vi "test NtripClient_mount point only.vi"() -> ()   [LabVIEW 2019]
uses:
  Ctrl/Ntrip_Account_db.ctl
panel:
  out "에러 출력 2":errorcluster caption="에러 출력"
  in  "탭 컨트롤":enum32{"Main", "ref", "wireshark capture"}(tab)
  in  "Mount points":u16(ring) items=["SONP-RTCM32", "GANS-RTCM32", "GUMC-RTCM32", "DBON-RTCM32", "YONS-RTCM23", "SONP-RTCM23", "GUMC-RTCM23", "GANS-RTCM31", "YONS-CMRx", "SONP-RTCM31", "GUMC-RTCM31", "GANS-RTCM23", "DBON-RTCM23", "DBON-RTCM31", "YONS-RTCM31", "YONS-RTCM32-M5", "VRS-RTCM32-M5", "VRS-RTCM31", "VRS-CMRx", "VRS-CMRplus"]
  out "mount points":string[](array[string])
  out "링 텍스트.텍스트":string
  in  "Current Ntrip account":T1={"address"="gnss.eseoul.go.kr", "port "=2101, "id"="seoul", "pwd"="seoul", "ref pt"="YONS-RTCM32-M5"}
  in  "read bytes":i32=10000
  out "데이터 출력":string
  out "s? t:f":string
  # "fkp.ngii.go.kr"
  # "Test Ntrip Client"
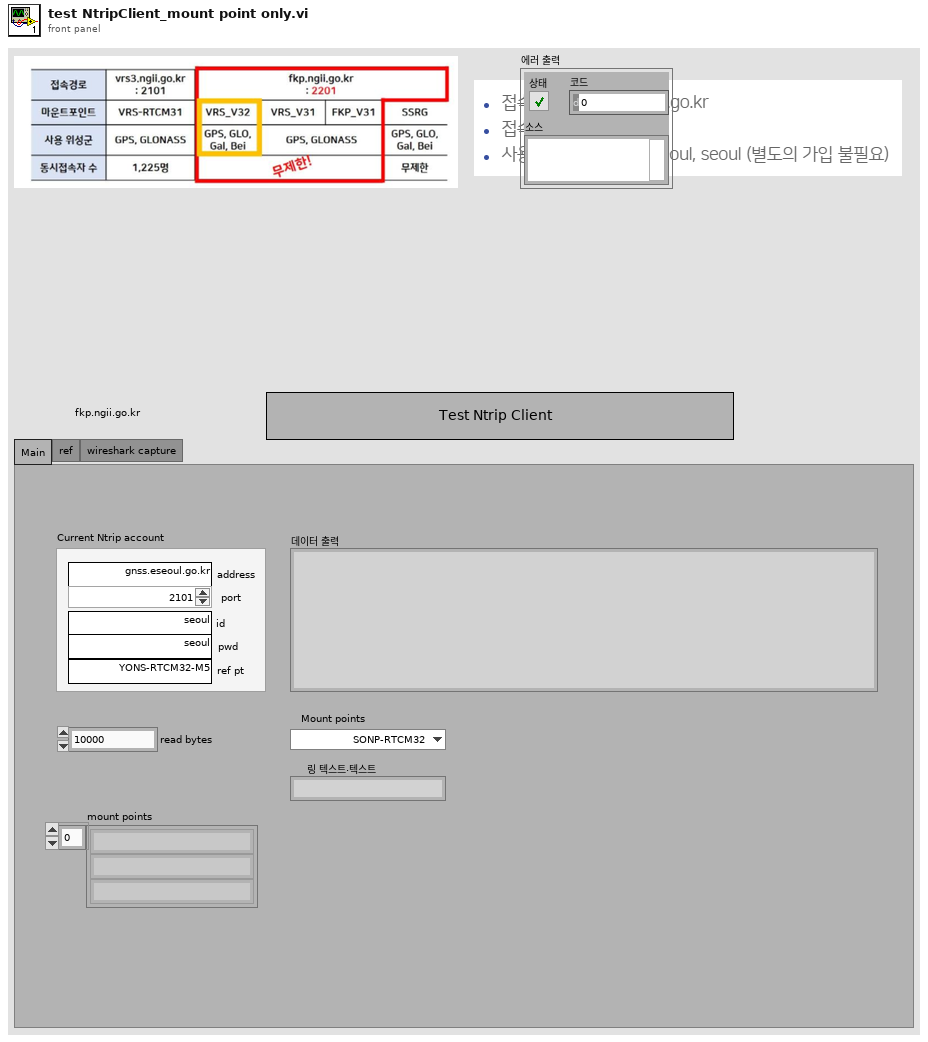
[diagram p1: front panel]
types:
  T1 = typedef "Ntrip_Account_db.ctl" = cluster{"address":string, "port ":u16, "id":string, "pwd":string, "ref pt":string}
  T2 = enum16{"Standard", "Buffered", "CRLF", "Immediate"}
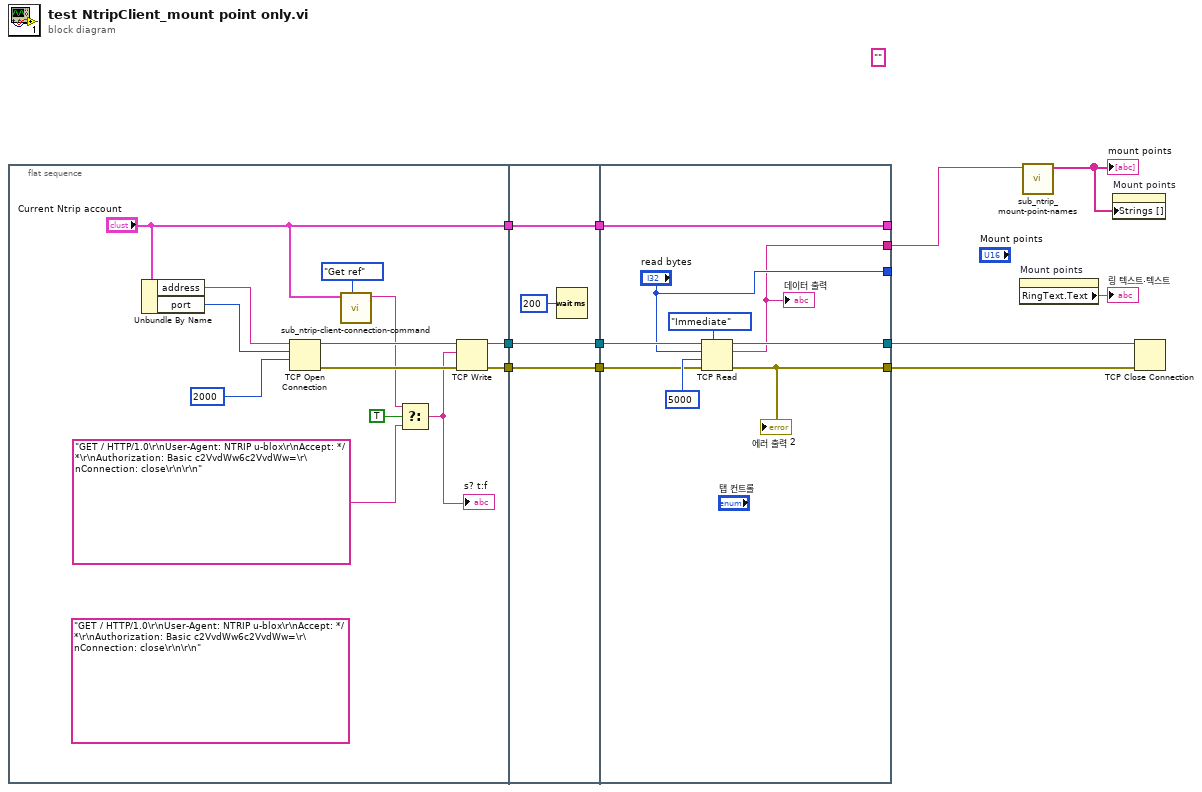
[diagram p0: block diagram]
diagram:
  (unwired) ""
  n1 = flat-sequence {
    tunnel: [w22] -> w11
    tunnel: [w21] -> w10
    tunnel: ["Current Ntrip account"] -> w9
    tunnel: w11 -> [w28]
    tunnel: w10 -> [w27]
    tunnel: w9 -> [w25]
    tunnel: [w28] -> w8
    tunnel: [w27] -> w7
    tunnel: [w25] -> w6
    tunnel: [w37] -> _
    tunnel: [w34] -> w5
    tunnel: [w31] -> w4
    tunnel: w8 -> [w32]
    tunnel: w7 -> [w33]
    tunnel: w6 -> [w37]
    tunnel: ["read bytes"] -> _
    tunnel: [w29] -> w1
    frame #0 {
      (unwired) "GET / HTTP/1.0\r\nUser-Agent: NTRIP u-blox\r\nAccept: */*\r\nAuthorization: Basic c2VvdWw6c2VvdWw=\r\nConnection: close\r\n\r\n" ("ascii 2")
      n2 = Unbundle By Name("Current Ntrip account") -> ("address"=w18:string, "port"=w17:u16)
      n3 = TCP Open Connection(address=w18, remote port or service name=w17, timeout ms (60000)=2000) -> (connection ID=w23:refnum<k5>, error out=w20:errorcluster)  [unwired: 2 in]
      n4 = call "sub_ntrip-client-connection-command.vi"("cmd"=enum16{"Get ref", "Get rtcm"}."Get ref", "Current Ntrip account"="Current Ntrip account") -> ("hex"=w14:string)  [unwired: 9 in]
      n5 = Select(t=w14, s=TRUE, f="GET / HTTP/1.0\r\nUser-Agent: NTRIP u-blox\r\nAccept: */*\r\nAuthorization: Basic c2VvdWw6c2VvdWw=\r\nConnection: close\r\n\r\n" ("ascii 2")) -> (s? t:f=w12:string)
      "s? t:f" <- w12
      n6 = TCP Write(connection ID=w23, data in=w12, error in (no error)=w20) -> (connection ID out=w21:refnum<k5>, error out=w22:errorcluster)  [unwired: 1 in, 1 out]
    }
    frame #1 {
      n7 = Wait (ms)(milliseconds to wait=u32 200) -> ()  [unwired: 1 out]
    }
    frame #2 {
      n8 = TCP Read(connection ID=w33, bytes to read="read bytes", error in (no error)=w32, 7:T2."Immediate" ("mode (standard)"), 9:5000 ("타임아웃 ms (25000)")) -> (connection ID out=w34:refnum<k5>, data out=w29:string, error out=w31:errorcluster)
      "데이터 출력" <- w29
      "에러 출력 2" <- w31
    }
  }
  n9 = property on="Mount points" class="Ring (strict)"() -> ("RingText.Text"=→"링 텍스트.텍스트":string)  [unwired: 2 in, 2 out]
  n10 = call "sub_ntrip_mount-point-names.vi"("ntrip str"=w1) -> ("mount points"=w3:string[])  [unwired: 10 in]
  "mount points" <- w3
  n11 = property on="Mount points" class="Ring (strict)"("Strings []"=w3) -> ()  [unwired: 2 in, 2 out]
  n12 = TCP Close Connection(connection ID=w5, error in (no error)=w4) -> ()  [unwired: 1 in, 2 out]
